vi "Teleop.vi"(10 "Match Info":T1={"Autonomous Elapsed Seconds"=0.0, "TeleOp Elapsed Seconds"=0.0, "Disabled Elapsed Seconds"=0.0, "Visited Autonomous"=FALSE, "Visited TeleOp"=FALSE, "Visited Disabled"=FALSE, "Autonomous Settings"={"Autonomous Style"=enum."Independent", "VI Refnum"=refnum}}, 11 "Call Context":T2) -> ()   [LabVIEW 2017]
doc: "This VI is called for each TeleOp packet received from the DS where the robot is not disabled. It is often used to read from the joysticks and update I/O or to update setpoints for timed control loops. It should complete and return within 20 milliseconds or it may miss DS packets."
uses:
  <vilib>/Rock Robotics/WPI/DriverStation/WPI_DriverStationDerivedRobotMode.ctl
  <vilib>/Rock Robotics/WPI/DriverStation/WPI_DriverStationMatch Info.ctl
  <vilib>/Rock Robotics/WPI/Solenoid/WPI_SolenoidValue.ctl
  <vilib>/Rock Robotics/WPI/Utilities/WPI_GetSetVariantRefNum.vi
  <vilib>/Rock Robotics/Network Tables/NT Write Boolean Array.vi
  <vilib>/Rock Robotics/Network Tables/NT Read Boolean.vi
  <vilib>/Rock Robotics/Network Tables/NT Read Number.vi
  <vilib>/Rock Robotics/Network Tables/NT Write Number.vi
  <vilib>/Rock Robotics/Network Tables/NT Write Numeric Array.vi
  <vilib>/Rock Robotics/WPI/RobotDrive/WPI_RobotDriveArcadeDrive_Standard(NoSaturation).vi
  <vilib>/Rock Robotics/WPI/Solenoid/WPI_SolenoidSetEnum.vi
panel:
  out "Sample Slider 0":dbl(slide) scale=0.0..5.0
  out "Sample Boolean 1":bool
  out "Sample Boolean 0":bool
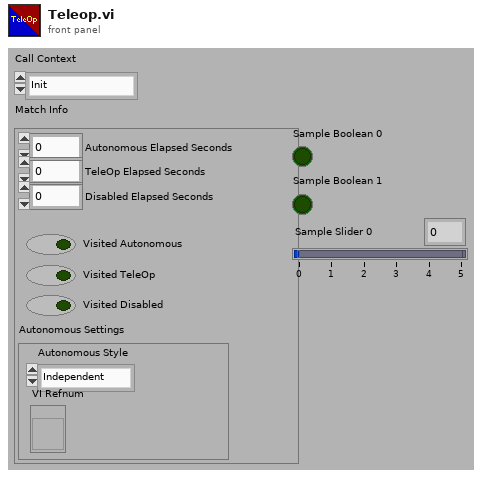
[diagram p1: front panel]
types:
  T1 = typedef "WPI_DriverStationMatch Info.ctl" = cluster{"Autonomous Elapsed Seconds":dbl, "TeleOp Elapsed Seconds":dbl, "Disabled Elapsed Seconds":dbl, "Visited Autonomous":bool, "Visited TeleOp":bool, "Visited Disabled":bool, "Autonomous Settings":cluster{"Autonomous Style":enum16{"Iterative", "Independent"}, "VI Refnum":refnum<vi>}}
  T2 = typedef "WPI_DriverStationDerivedRobotMode.ctl" = enum16{"Init", "Execute", "Stop"}
  T3 = typedef "WPI_SolenoidValue.ctl" = enum16{"Off", "On", "Forward", "Reverse"}
  T4 = typedef "WPI_JoystickDevRef.ctl" = cluster{"Device":T5}
  T5 = typedef "WPI_JoystickDeviceEnum.ctl" = enum16{"USB 0", "USB 1", "USB 2", "USB 3", "USB 4", "USB 5"}
  T6 = cluster{"Axes[0]":dbl, "Axes[1]":dbl, "Axes[2]":dbl, "Axes[3]":dbl, "Axes[4]":dbl, "Axes[5]":dbl, "Axes[6]":dbl, "Axes[7]":dbl, "Axes[8]":dbl}
  T7 = cluster{"Buttons[0]":bool, "Buttons[1]":bool, "Buttons[2]":bool, "Buttons[3]":bool, "Buttons[4]":bool, "Buttons[5]":bool, "Buttons[6]":bool, "Buttons[7]":bool, "Buttons[8]":bool}
  T8 = typedef "WPI_SolenoidDevRef.ctl" = cluster{"DevStatus":errorcluster, "Pneumatics Control Module":u8, "Forward Solenoid Channel":T9, "Reverse Solenoid Channel":T9}
  T9 = typedef "WPI_SolenoidChannel.ctl" = enum8{"Solenoid 0", "Solenoid 1", "Solenoid 2", "Solenoid 3", "Solenoid 4", "Solenoid 5", "Solenoid 6", "Solenoid 7", "Invalid"}
  T10 = typedef "WPI_MotorControlDeviceRef.ctl" = cluster{"DeviceStatus":errorcluster, "Type":T11, "PWM":cluster{"PWM Channel":T12, "DeadBand":T13}, "CAN":cluster{"Device Number":u8, "SetOutput VI Ref":variant, "GetOutput VI Ref":variant, "Enable VI Ref":variant, "Disable VI Ref":variant, "Data":variant}, "Invert":bool, "DIO PWM":cluster{"PWM \"Enable\" Channel":T12, "DIOChannel":T14, "PWM Rate":dbl}}
  T11 = typedef "WPI_MotorControlType.ctl" = enum16{"PWM", "CAN", "DIO PWM"}
  T12 = typedef "FPGA_DIOPWMChannel.ctl" = enum8{"PWM 0", "PWM 1", "PWM 2", "PWM 3", "PWM 4", "PWM 5", "PWM 6", "PWM 7", "PWM 8", "PWM 9", "PWM MXP 0", "PWM MXP 1", "PWM MXP 2", "PWM MXP 3", "PWM MXP 4", "PWM MXP 5", "PWM MXP 6", "PWM MXP 7", "PWM MXP 8", "PWM MXP 9", "Invalid"}
  T13 = typedef "WPI_PWMDeadband.ctl" = cluster{"Name":string, "maxPositivePwm":i32, "minPositivePwm":i32, "centerPwm":i32, "maxNegativePwm":i32, "minNegativePwm":i32, "angularRange":u16}
  T14 = typedef "FPGA_DIOChannel.ctl" = enum8{"DIO 0", "DIO 1", "DIO 2", "DIO 3", "DIO 4", "DIO 5", "DIO 6", "DIO 7", "DIO 8", "DIO 9", "DIO MXP 0", "DIO MXP 1", "DIO MXP 2", "DIO MXP 3", "DIO MXP 4", "DIO MXP 5", "DIO MXP 6", "DIO MXP 7", "DIO MXP 8", "DIO MXP 9", "DIO MXP 10", "DIO MXP 11", "DIO MXP 12", "DIO MXP 13", "DIO MXP 14", "DIO MXP 15", "SPI Port CS1", "SPI Port CS2", "SPI Port CS3", "SPI Port MISO", "SPI Port MOSI", "Invalid"}
  T15 = typedef "WPI_RobotDriveDevRef.ctl" = cluster{"DevStatus":errorcluster, "Motors[]":T10[], "Square Inputs":bool, "Max Output":dbl}
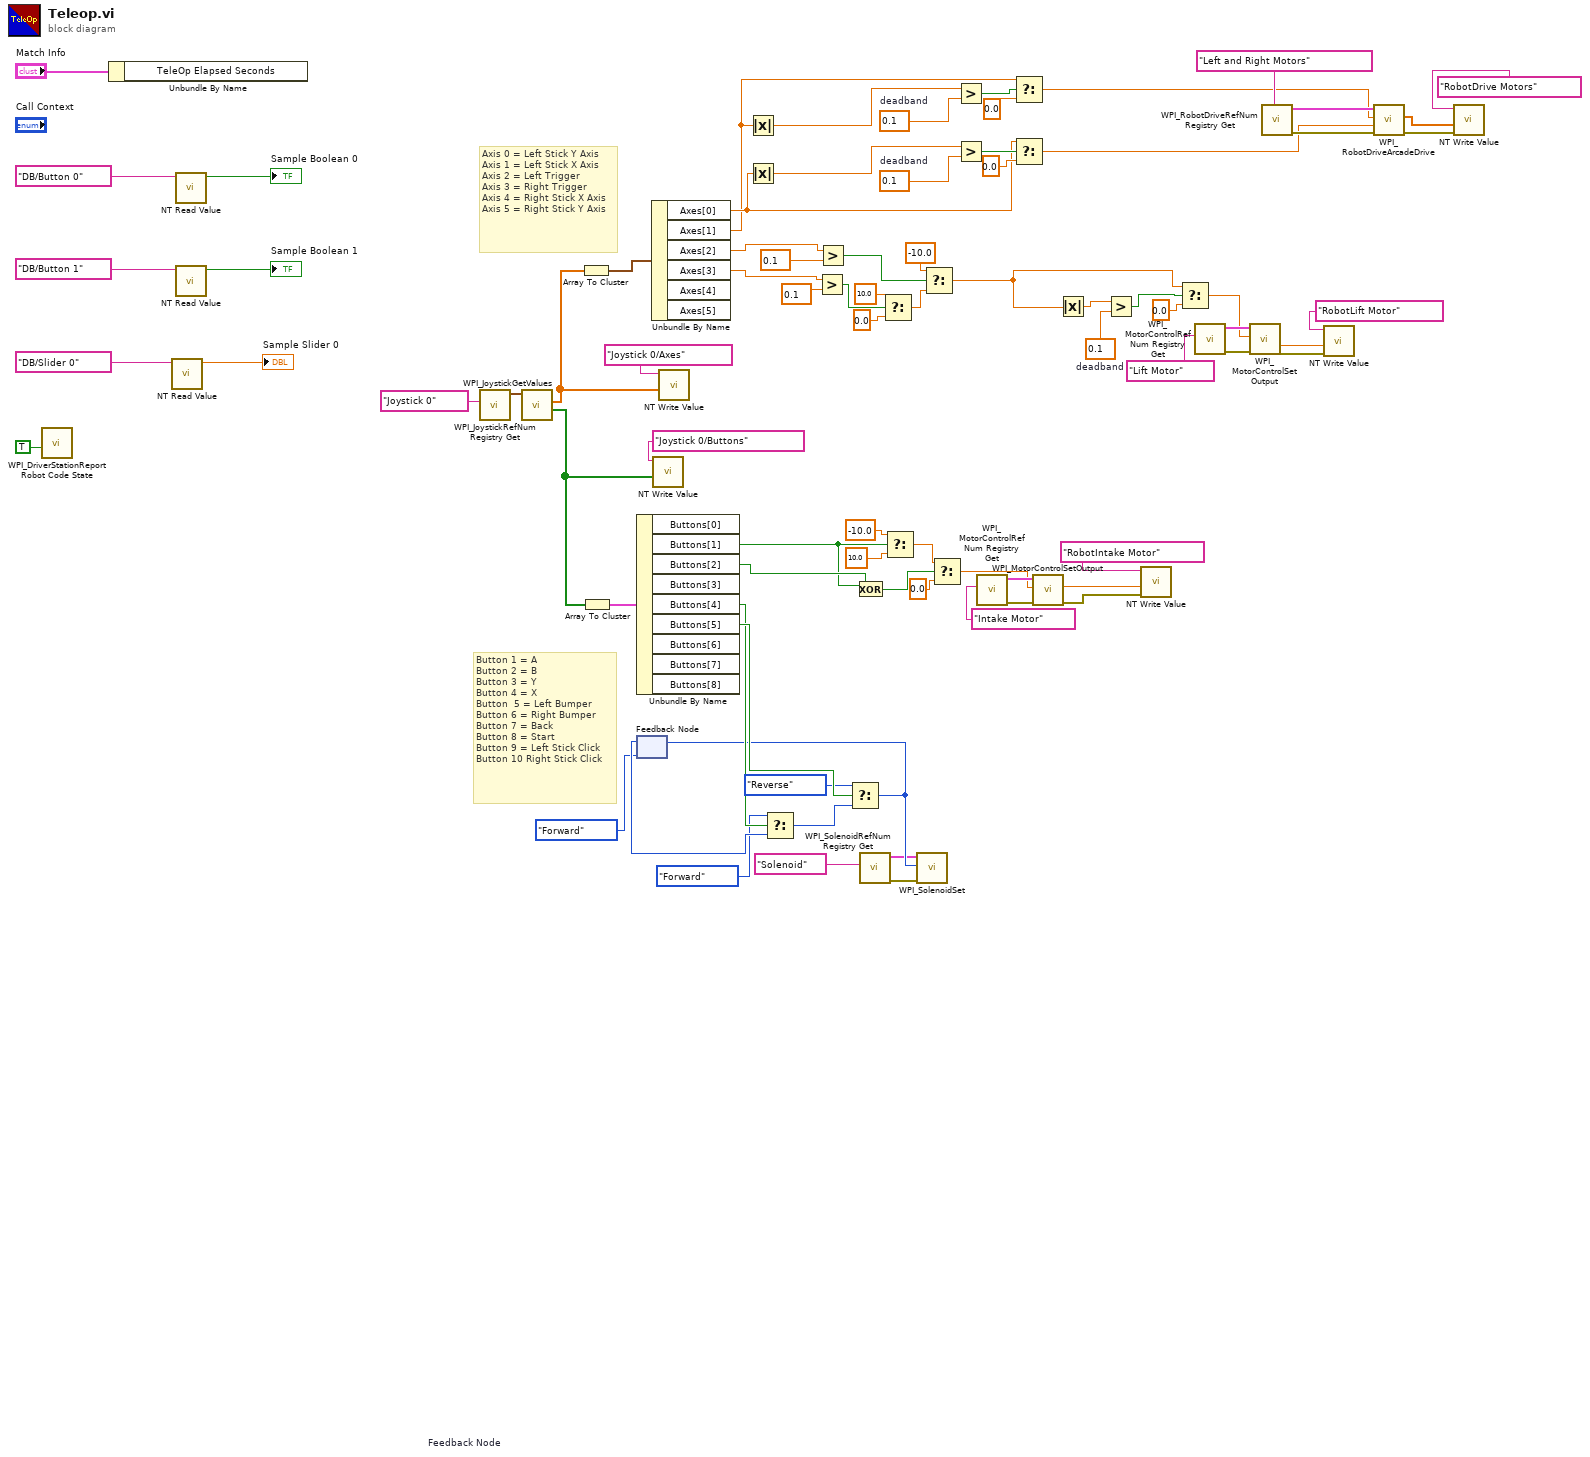
[diagram p0: block diagram]
diagram:
  w12 = 0.1  # deadband
  w17 = 0.1  # deadband
  w22 = 0.1  # deadband
  # "Axis 0 = Left Stick Y Axis\nAxis 1 = Left Stick X Axis\nAxis 2 = Left Trigger\nAxis 3 = Right Trigger\nAxis 4 = Right Stick X Axis\nAxis 5 = Right Stick Y Axis"
  # "Button 1 = A\nButton 2 = B\nButton 3 = Y\nButton 4 = X\nButton  5 = Left Bumper\nButton 6 = Right Bumper\nButton 7 = Back\nButton 8 = Start\nButton 9 = Left Stick Click\nButton 10 Right Stick Click"
  n1 = call <vilib>:"WPI_DriverStationReport Robot Code State.vi"("TeleOp"=TRUE ("Autonomous")) -> ()  [unwired: 10 in, 1 out]
  n2 = Unbundle By Name("Match Info") -> ()  [unwired: 1 out]
  n3 = call-poly <vilib>:"NT Read Value.vi"("Name"="DB/Slider 0" ("refnum name")) -> ("Numeric"=→"Sample Slider 0":dbl)  [unwired: 9 in, 1 out]
  n4 = call-poly <vilib>:"NT Read Value.vi"("Name"="DB/Button 0" ("refnum name")) -> ("Boolean"=→"Sample Boolean 0":bool)  [unwired: 9 in, 1 out]
  n5 = call-poly <vilib>:"NT Read Value.vi"("Name"="DB/Button 1" ("refnum name")) -> ("Boolean"=→"Sample Boolean 1":bool)  [unwired: 9 in, 1 out]
  n6 = call <vilib>:"WPI_JoystickRefNum Registry Get.vi"("refnum name"="Joystick 0") -> ("JoystickDevRef"=w77:T4)  [unwired: 1 in, 9 out]
  n7 = call <vilib>:"WPI_JoystickGetValues.vi"("JoystickDevRef"=w77) -> ("Buttons"=w64:bool[], "Axes"=w66:dbl[])  [unwired: 6 in, 3 out]
  n8 = Array To Cluster(array=w66) -> (cluster=w65:T6)
  n9 = Array To Cluster(array=w64) -> (cluster=w63:T7)
  n10 = Unbundle By Name(w63) -> ("Buttons[1]"=w61:bool, "Buttons[2]"=w62:bool, "Buttons[4]"=w59:bool, "Buttons[5]"=w60:bool)  [unwired: 5 out]
  n11 = feedback #1 "Feedback Node"(WPI_SolenoidValue."Forward" ("Value")) -> (w38:T3)
  n12 = Unbundle By Name(w65) -> ("Axes[0]"=w19:dbl, "Axes[1]"=w14:dbl, "Axes[2]"=w2:dbl, "Axes[3]"=w1:dbl)  [unwired: 2 out]
  n13 = call-poly <vilib>:"NT Write Value.vi"("Boolean Array"=w64, "Name"="Joystick 0/Buttons") -> ()  [unwired: 9 in, 1 out]
  n14 = call-poly <vilib>:"NT Write Value.vi"("Numeric Array"=w66, "Name"="Joystick 0/Axes") -> ()  [unwired: 9 in, 1 out]
  n15 = Absolute Value(x=w14) -> (abs(x)=w18:dbl)
  n16 = Absolute Value(x=w19) -> (abs(x)=w23:dbl)
  n17 = Select(t=WPI_SolenoidValue."Forward" ("Value"), s=w59, f=w38) -> (s? t:f=w32:T3)
  n18 = Greater?(x=w1, y=0.1) -> (0:w49:bool)
  n19 = Greater?(x=w2, y=0.1) -> (0:w48:bool)
  n20 = Select(t=WPI_SolenoidValue."Reverse" ("Value"), s=w60, f=w32) -> (s? t:f=w36:T3)
  n21 = feedback-in #1(w36) -> ()
  n22 = Exclusive Or(1:w62, 2:w61) -> (0:w45:bool)
  n23 = call <vilib>:"WPI_SolenoidRefNum Registry Get.vi"("refnum name"="Solenoid") -> ("error out"=w24:errorcluster, "SolenoidDevRef"=w33:T8)  [unwired: 9 in]
  n24 = Select(t=10.0, s=w49, f=0.0) -> (s? t:f=w54:dbl)
  n25 = Select(t=-10.0, s=w61, f=10.0) -> (s? t:f=w46:dbl)
  n26 = call-poly <vilib>:"WPI_SolenoidSet.vi"("error in (no error)"=w24, "Value"=w36, "SolenoidDevRef"=w33) -> ()  [unwired: 7 in, 2 out]
  n27 = Select(t=-10.0, s=w48, f=w54) -> (s? t:f=w9:dbl)
  n28 = Select(t=w46, s=w45, f=0.0) -> (s? t:f=w7:dbl)
  n29 = Greater?(x=w18, y=w17) -> (0:w16:bool)
  n30 = Greater?(x=w23, y=w22) -> (0:w21:bool)
  n31 = call <vilib>:"WPI_MotorControlRefNum Registry Get.vi"("refnum name"="Intake Motor") -> ("error out"=w25:errorcluster, "MotorControlDevRef"=w43:T10)  [unwired: 9 in]
  n32 = Select(t=w14, s=w16, f=0.0) -> (s? t:f=w5:dbl)
  n33 = Select(t=w19, s=w21, f=0.0) -> (s? t:f=w4:dbl)
  n34 = call <vilib>:"WPI_MotorControlSetOutput.vi"("error in (no error)"=w25, "Output"=w7, "MotorControlDevRef"=w43) -> ("error out"=w26:errorcluster, "Motor Output"=w44:dbl)  [unwired: 6 in, 1 out]
  n35 = Absolute Value(x=w9) -> (abs(x)=w13:dbl)
  n36 = Greater?(x=w13, y=w12) -> (0:w11:bool)
  n37 = call-poly <vilib>:"NT Write Value.vi"("error in"=w26, "Numeric"=w44, "Name"="RobotIntake Motor") -> ()  [unwired: 8 in, 1 out]
  n38 = Select(t=w9, s=w11, f=0.0) -> (s? t:f=w8:dbl)
  n39 = call <vilib>:"WPI_MotorControlRefNum Registry Get.vi"("refnum name"="Lift Motor") -> ("error out"=w27:errorcluster, "MotorControlDevRef"=w57:T10)  [unwired: 9 in]
  n40 = call <vilib>:"WPI_MotorControlSetOutput.vi"("error in (no error)"=w27, "Output"=w8, "MotorControlDevRef"=w57) -> ("error out"=w28:errorcluster, "Motor Output"=w56:dbl)  [unwired: 6 in, 1 out]
  n41 = call <vilib>:"WPI_RobotDriveRefNum Registry Get.vi"("refnum name"="Left and Right Motors") -> ("error out"=w30:errorcluster, "RobotDriveDevRef"=w79:T15)  [unwired: 1 in, 8 out]
  n42 = call-poly <vilib>:"NT Write Value.vi"("error in"=w28, "Numeric"=w56, "Name"="RobotLift Motor") -> ()  [unwired: 8 in, 1 out]
  n43 = call-poly <vilib>:"WPI_RobotDriveArcadeDrive.vi"("error in (no error)"=w30, "Y axis value"=w4, "X axis value"=w5, "RobotDriveDevRef"=w79) -> ("error out"=w29:errorcluster, "Motor Values"=w68:dbl[])  [unwired: 5 in, 1 out]
  n44 = call-poly <vilib>:"NT Write Value.vi"("error in"=w29, "Numeric Array"=w68, "Name"="RobotDrive Motors") -> ()  [unwired: 8 in, 1 out]
